vi "GPS_usb 파싱.vi"() -> ()   [LabVIEW 2020]
uses:
  <vilib>/Instr/_visa.llb/VISA Configure Serial Port (Instr).vi
panel:
  in  "탭 컨트롤":T1(tab)
  out "로그파일 데이터":cluster{"all rows":dbl[], "all rows":dbl[]}(graph)
  out "보간 데이터":cluster{"all rows":dbl[], "all rows":dbl[]}(graph)
  out "거리값 설정 데이터":cluster{"all rows":dbl[], "all rows":dbl[]}(graph)
  in  "로그 파일 경로":path
  in  "배수 설정":i32
  in  "거리 값":dbl=1.0 format="%#_13g"
  in  "로그 인덱스 선택(0)":i32
  in  "로그 인덱스 선택(1)":i32=1
  in  "보간 방법":i32(ring)=1 items=["최근접", "선형", "스플라인", "3차 에르미트", "라그랑지"]
  out "RMC":T2 {"Checksum" format="%x"}
  out "GGA":T3 {"Checksum" format="%x"}
  out "VTG":T4 {"Checksum" format="%x"}
  out "구좌표플롯":cluster{"배열":dbl[], "배열":dbl[]}(graph)
  out "평면좌표플롯":cluster{"배열":dbl[], "배열":dbl[]}(graph)
  out "버퍼 읽기":string
  out "도(Lat)":string
  out "도(Long)":string
  out "도분초(Long)":string
  out "도분초(Lat)":string
  out "Y(E)":dbl format="%#.6g"
  out "X(N)":dbl format="%#.6g"
  out "에러 출력":errorcluster
  in  "정지":bool
  in  "VISA name":refnum<visa-resource-name> caption="VISA 리소스 이름"
  in  "baud rate  2":u32=9600 caption="보 전송속도(9600)"
  in  "timeout":u32=10000 caption="타임아웃(10sec)"
  in  "에러 입력(에러 없음)":errorcluster
  out "결과 조향값":dbl format="%#_13g"
  in  "Ld":dbl
  in  "다음wp X값":dbl format="%#_13g"
  in  "GPS X값":dbl format="%#_13g"
  in  "다음wp Y값":dbl format="%#_13g"
  in  "GPS Y값":dbl format="%#_13g"
  in  "GPS 헤딩값":dbl format="%#_13g"
  in  "축거(m)":dbl=1.04 format="%#_13g"
  in  "시리얼 루프 정지":bool
  out "Receive Data":T5
  in  "E-Stop":enum8{"정상", "긴급정지"}(ring)
  in  "transmit Data":T6
  in  "시리얼 포트 설정":refnum<visa-resource-name> caption="VISA 리소스 이름"
  in  "baud rate":u32=9600 caption="보 전송속도(9600)"
  in  "timeout (100)":u32=10000 caption="타임아웃(10sec)"
  out "Lidar":cluster{"배열":dbl[], "배열":dbl[]}(graph)
  out "time stamp + factory":string
  in  "Lidar 정지":bool
  out "Mixed Signal Graph":cluster{dbl[], dbl[]}[](graph)
  out "Mixed Signal Graph 2":cluster{"array":dbl[], "array":dbl[]}[](graph)
  in  "점 개수":i32
  in  "사각형 크기 설정값":dbl
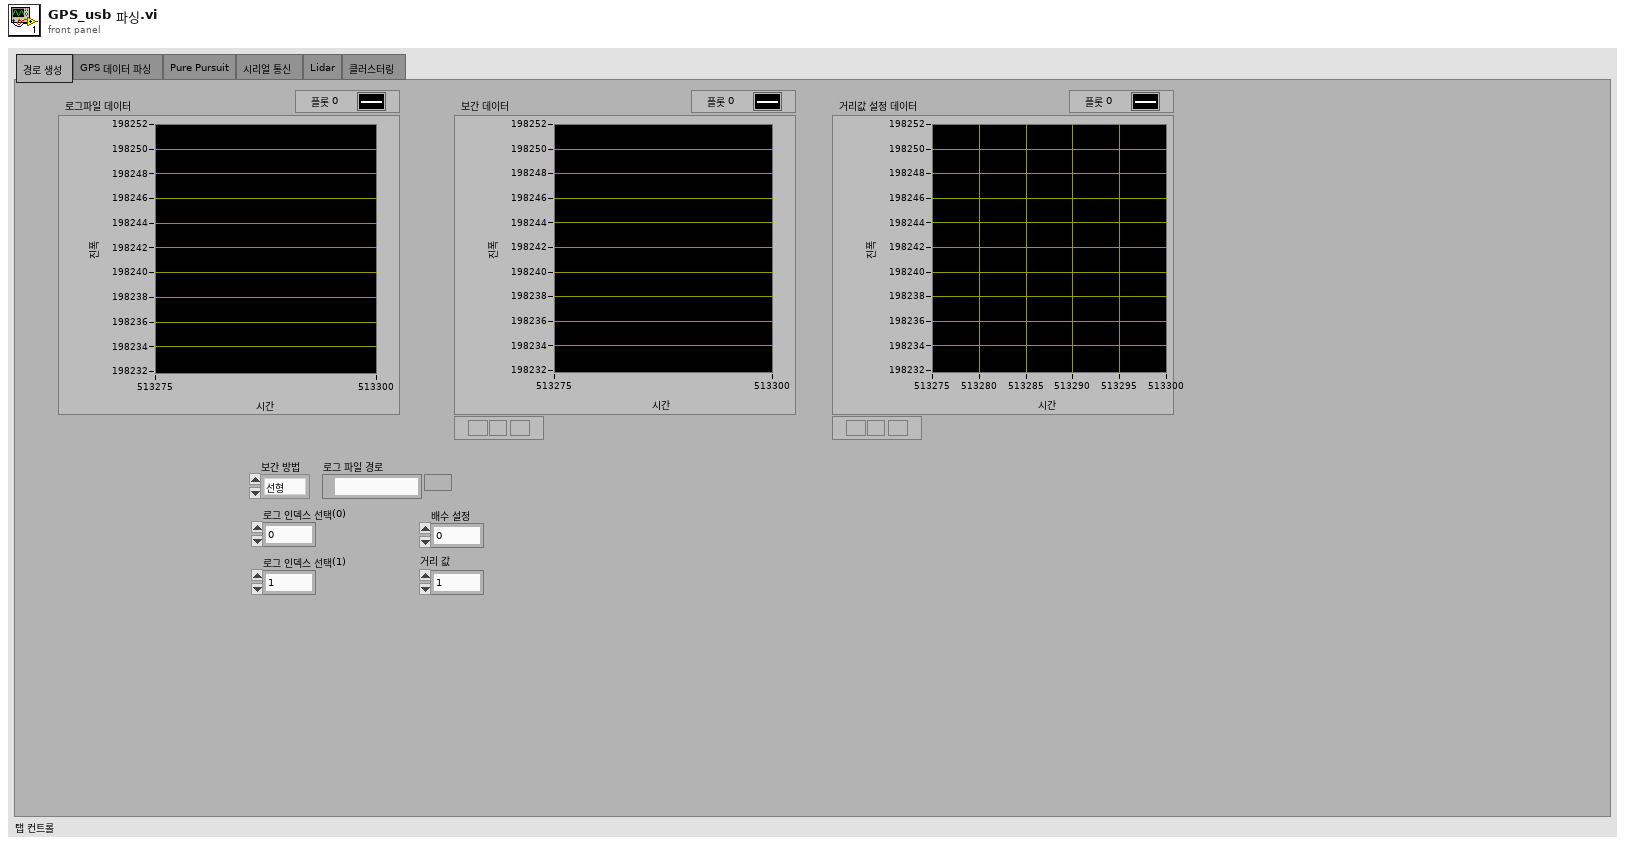
[diagram p1: front panel]
types:
  T1 = enum32{"경로 생성", "GPS 데이터 파싱", "Pure Pursuit", "시리얼 통신", "Lidar", "클러스터링"}
  T2 = cluster{"UTC time":dbl, "Status":string, "Latitude":dbl, "N/S Indicator":string, "Longitude":dbl, "E/W Indicator":string, "Speed":dbl, "Degrees":dbl, "UTC date":dbl, "Null":string, "Null 2":string, "Null 3":string, "Null 4":string, "Checksum":i32}
  T3 = cluster{"UTC time":dbl, "Latitude":dbl, "N/S Indicator":string, "Longitude":dbl, "E/W Indicator":string, "Position FIx":i32, "Satelites Used":i32, "HDOP":dbl, "Altitude":dbl, "Altitude Units":string, "empty":string, "empty":string, "empty":string, "Checksum":u8}
  T4 = cluster{"Course":dbl, "Reference":string, "Course in degrees":dbl, "Reference":string, "Speed":dbl, "Unit":string, "Speed":dbl, "K":string, "A":string, "Checksum":u8}
  T5 = cluster{"AorM":u8, "E-Stop":u8, "F_B":u8, "Speed":u16, "Steer":i16, "Brake":u8, "Encoder":u8, "Encoder2":u8, "Encoder3":u8, "Encoder4":u8, "ALIVE":u8, "ETX_0":u8, "ETX_1":u8}
  T6 = cluster{enum8{"Manual", "Auto"}, enum8{"전진", "중립", "후진"}, "Speed":u16, "Steer":i16, "Brake":u8}
  T7 = enum16{"open", "replace", "create", "open or create", "replace or create", "replace or create with confirmation"}
  T8 = cluster{"UTC time":dbl, "Status":string, "Latitude":dbl, "N/S Indicator":string, "Longitude":dbl, "E/W Indicator":string, "Speed":dbl, "Degrees":dbl, "UTC date":dbl, "Null":string, "Null 2":string, "Null 3":string, "Null 4":string, "Checksum":u8}
  T9 = cluster{"string array[0]":string, "string array[1]":string, "string array[2]":string, "string array[3]":string, "string array[4]":string, "string array[5]":string, "string array[6]":string, "string array[7]":string, "string array[8]":string, "string array[9]":string, "string array[10]":string, "string array[11]":string, "string array[12]":string}
  T10 = cluster{"string array[0]":string, "string array[1]":string, "string array[2]":string, "string array[3]":string, "string array[4]":string, "string array[5]":string, "string array[6]":string, "string array[7]":string, "string array[8]":string}
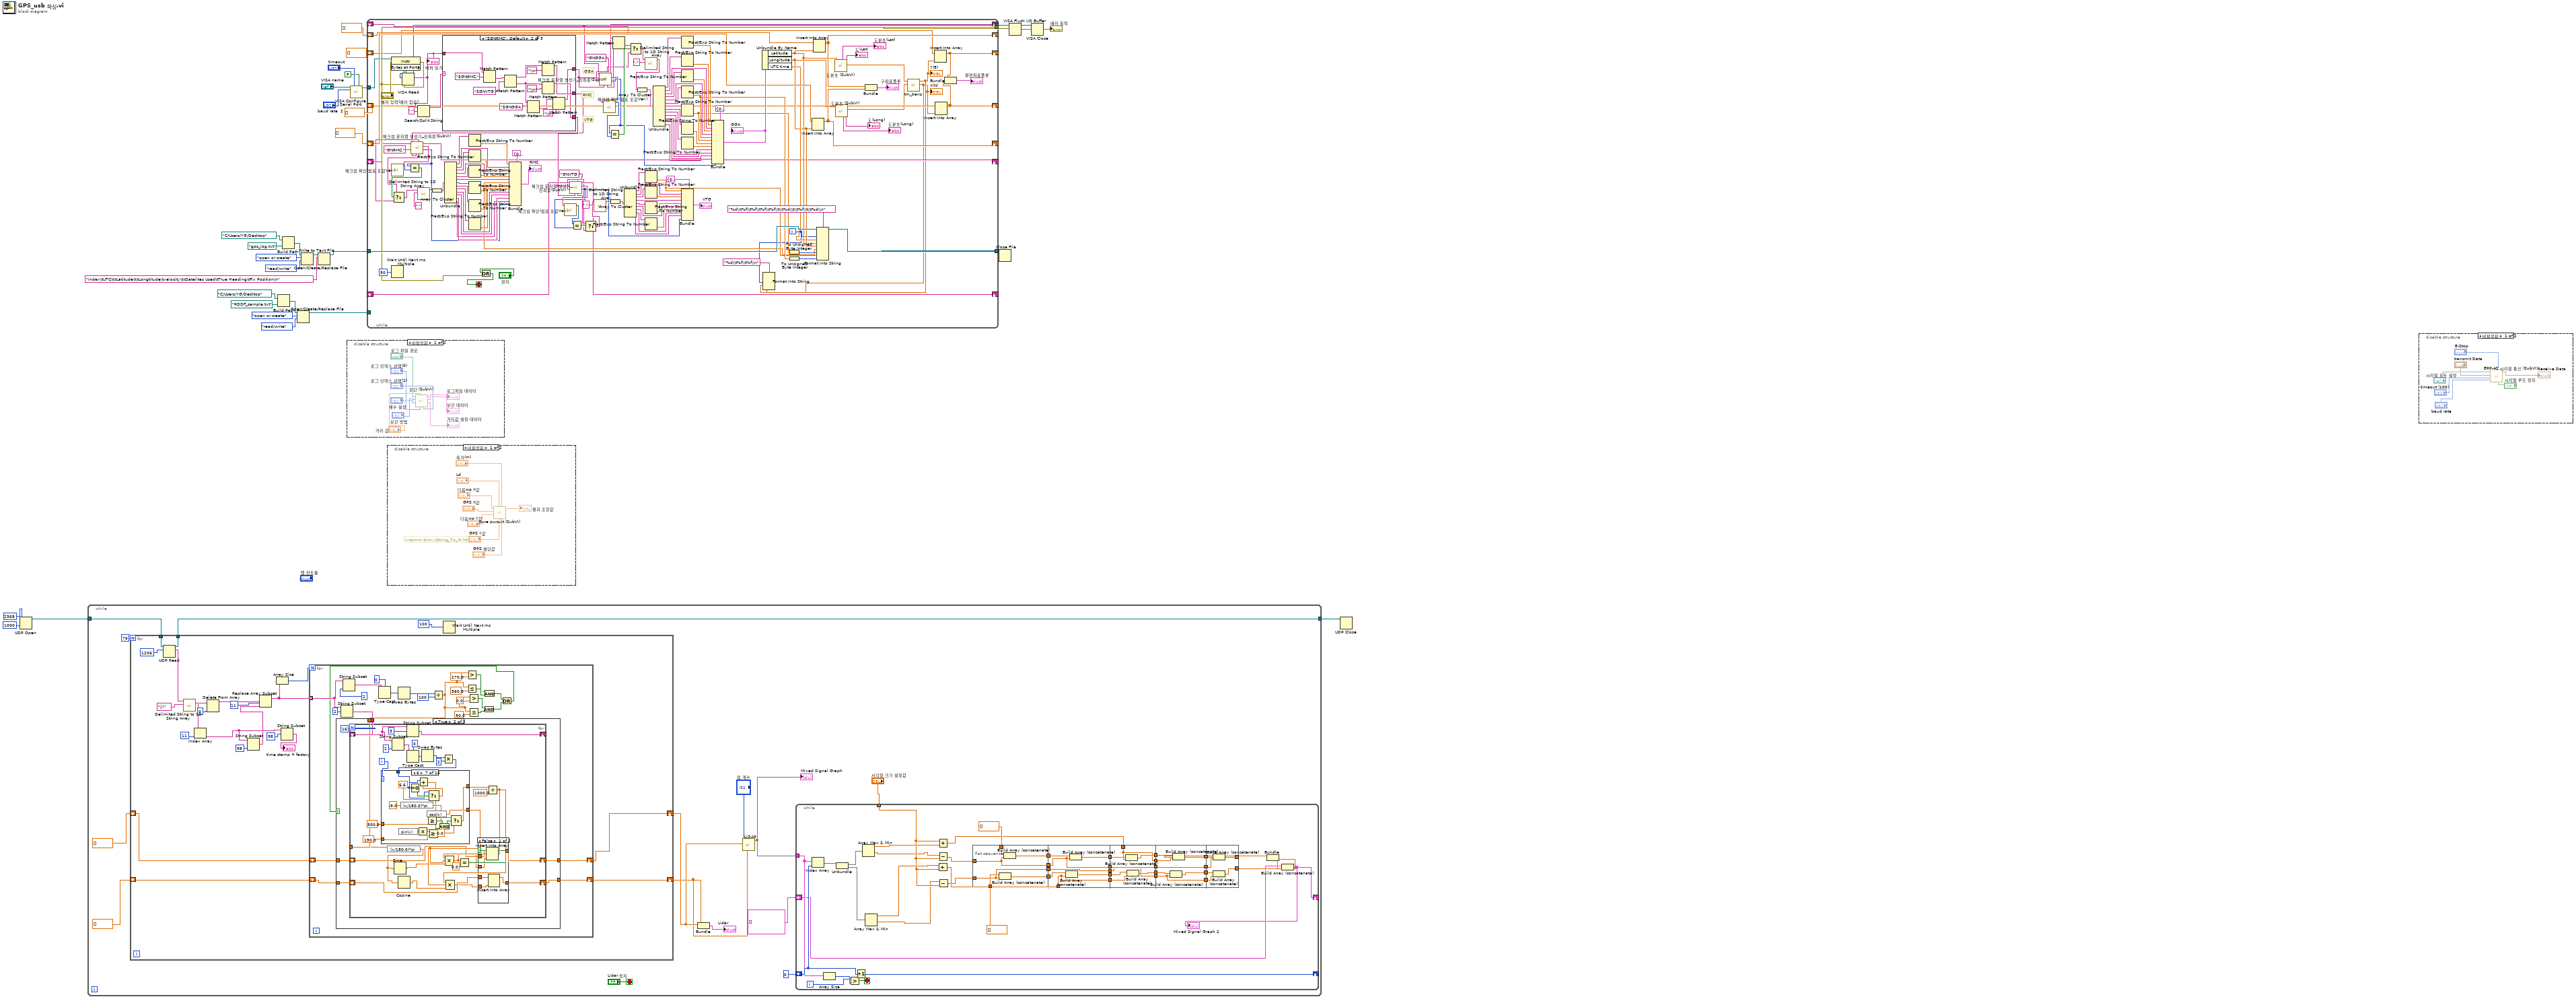
[diagram p0: block diagram]
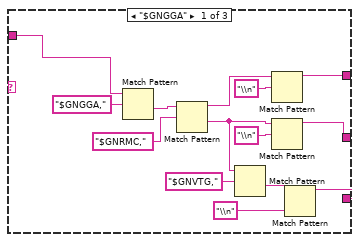
[diagram p2: hidden frame]
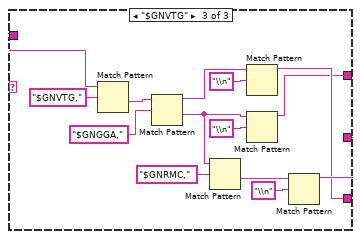
[diagram p3: hidden frame]
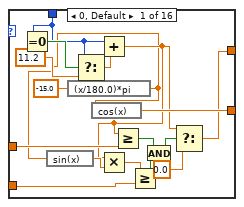
[diagram p6: hidden frame]
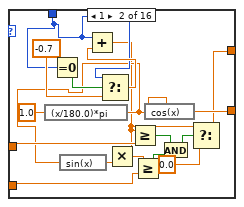
[diagram p7: hidden frame]
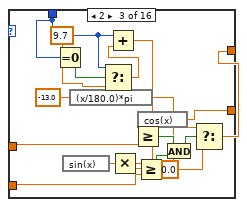
[diagram p8: hidden frame]
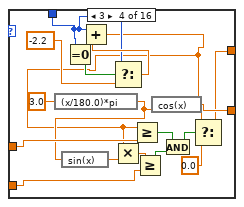
[diagram p9: hidden frame]
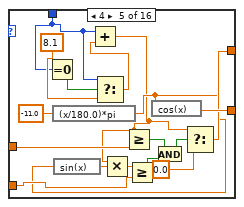
[diagram p10: hidden frame]
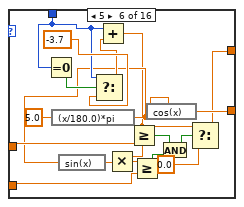
[diagram p11: hidden frame]
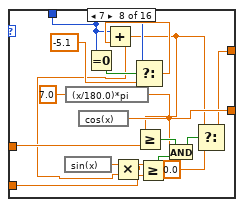
[diagram p12: hidden frame]
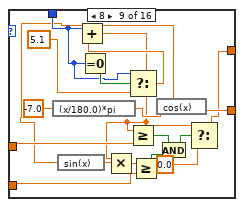
[diagram p13: hidden frame]
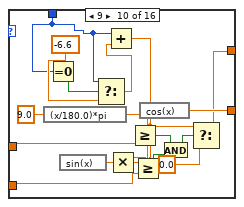
[diagram p14: hidden frame]
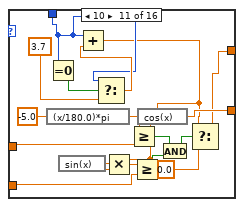
[diagram p15: hidden frame]
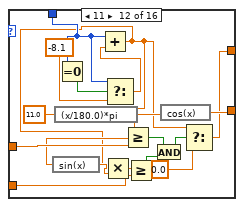
[diagram p16: hidden frame]
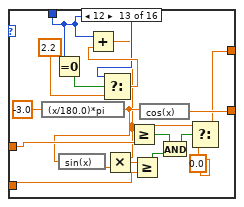
[diagram p17: hidden frame]
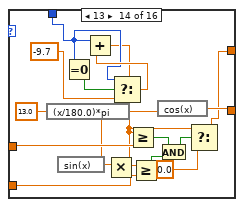
[diagram p18: hidden frame]
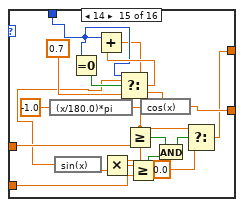
[diagram p19: hidden frame]
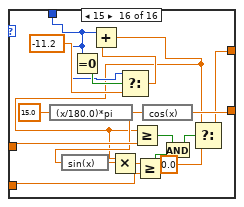
[diagram p20: hidden frame]
diagram:
  n1 = UDP Open(9:1000 ("타임아웃 ms (25000)"), 11:u16 2368 ("포트")) -> (port=w31:refnum<k16>)  [unwired: 3 in, 2 out]
  n2 = while {
    tunnel: w31 -> [w45]
    tunnel: [w44] -> w30
    stop <- "Lidar 정지" stop-if-true
    n3 = for {
      N: 76 -> [_]
      shift-right: [w127] -> w39
      shift-left: dbl[] [] -> [w132]
      shift-right: [w126] -> w38
      shift-left: dbl[] [] -> [w133]
      tunnel: w45 -> [w130]
      tunnel: [w128] -> w44
      n4 = UDP Read(connection ID=w130, max size (548)=1206 ("최대 크기(548)")) -> (data out=w129:string, 3:w128:refnum<k16>)  [unwired: 2 in, 3 out]
      n5 = call <vilib>:"Delimited String to 1D String Array.vi"("delimiter"="ÿî", "delimited string"=w129) -> ("string array"=w145:string[])  [unwired: 9 in]
      n6 = Delete From Array(array=w145, index=0 ("인덱스")) -> (array with subset deleted=w142:string[])  [unwired: 1 in, 1 out]
      n7 = Index Array(array=w142, index=11 ("인덱스")) -> (element=w138:string)
      n8 = String Subset(string=w138, length (rest)=98 ("길이(나머지)")) -> (substring=w137:string)  [unwired: 1 in]
      n9 = Replace Array Subset(array=w142, new element=w137, index=11 ("인덱스")) -> (w135:string[])
      n10 = Array Size(array=w135) -> (size(s)=w134:i32)
      n11 = String Subset(string=w138, offset (0)=98 ("오프셋(0)")) -> (substring=→"time stamp + factory":string)  [unwired: 1 in]
      n12 = for {
        N: w134 -> [_]
        tunnel: w135 -> [w164] mode=indexing
        shift-right: [w162] -> w126
        shift-left: w133 -> [w160]
        shift-right: [w161] -> w127
        shift-left: w132 -> [w159]
        n13 = String Subset(string=w164, offset (0)=2 ("오프셋(0)")) -> (substring=w163:string)  [unwired: 1 in]
        n14 = String Subset(string=w164, length (rest)=2 ("길이(나머지)")) -> (substring=w170:string)  [unwired: 1 in]
        n15 = Type Cast(type=u16 0, x=w170) -> (*(type *) &x=w168:u16)
        n16 = Swap Bytes(anything=w168) -> (byte swapped=w167:u16)
        n17 = Divide(x=w167, y=u16 100) -> (x/y=w152:dbl)
        n18 = Greater?(x=w152, y=270.0) -> (0:w155:bool)
        n19 = Less Or Equal?(x=w152, y=360.0) -> (x <= y?=w156:bool)
        n20 = Greater?(x=w152, y=0.0) -> (0:w151:bool)
        n21 = Less Or Equal?(x=w152, y=90.0) -> (x <= y?=w150:bool)
        n22 = And(x=w151, y=w150) -> (x .and. y?=w147:bool)
        n23 = And(x=w155, y=w156) -> (x .and. y?=w148:bool)
        n24 = Or(x=w148, y=w147) -> (x .or. y?=w149:bool)
        n25 = case shown="True" w149 {
          tunnel: w163 -> [_ w179]
          tunnel: w152 -> [_ w178]
          tunnel: [w172 w177] -> w162
          tunnel: [w173 w176] -> w161
          tunnel: w160 -> [w172 w175]
          tunnel: w159 -> [w173 w174]
          frame False {
          }
          frame True {
            n26 = for {
              N: 16 -> [_]
              shift-right: [w207] -> _
              shift-left: w179 -> [w206]
              tunnel: w178 -> [w199]
              shift-right: [w186] -> w176
              shift-left: w174 -> [w187]
              shift-right: [w183] -> w177
              shift-left: w175 -> [w184]
              i -> [w193]
              n27 = expression code="(x/180.0)*pi"(w199) -> (w195:dbl)
              n28 = String Subset(string=w206, length (rest)=u16 2 ("길이(나머지)")) -> (substring=w203:string)  [unwired: 1 in]
              n29 = Sine(x=w195) -> (sin(x)=w194:dbl)
              n30 = Cosine(x=w195) -> (cos(x)=w196:dbl)
              n31 = String Subset(string=w206, offset (0)=3 ("오프셋(0)")) -> (substring=w207:string)  [unwired: 1 in]
              n32 = Type Cast(type=u16 0, x=w203) -> (*(type *) &x=w204:u16)
              n33 = Swap Bytes(anything=w204) -> (byte swapped=w201:u16)
              n34 = Multiply(x=w201, y=u16 2 ("x")) -> (x*y=w200:u16)
              n35 = case shown="6" w193 {
                tunnel: w200 -> [w229 w246 w263 w280 w297 w314 w331 w348 w365 w382 w399 w416 w433 w450 w467 w484]
                tunnel: [w225 w239 w257 w274 w291 w308 w324 w341 w359 w376 w393 w409 w426 w444 w461 w478] -> w191
                tunnel: [w233 w250 w267 w284 w301 w318 w335 w352 w369 w386 w403 w420 w437 w454 w471 w488] -> w197
                tunnel: 500.0 ("거리 값(min)") -> [w224 w242 w259 w276 w293 w310 w327 w344 w361 w378 w395 w412 w428 w446 w463 w480]
                tunnel: 150.0 ("높이 값(min)") -> [w223 w241 w258 w275 w292 w309 w326 w343 w360 w377 w394 w411 w429 w445 w462 w479]
                frame 0, Default {
                  n36 = Equal To 0?(x=w229) -> (x = 0?=w231:bool)
                  n37 = expression code="(x/180.0)*pi"(-15.0) -> (w219:dbl)
                  n38 = expression code="sin(x)"(w219) -> (w221:dbl)
                  n39 = Select(t=w229, s=w231, f=11.2 ("y")) -> (s? t:f=w232:dbl)
                  n40 = expression code="cos(x)"(w219) -> (w233:dbl)
                  n41 = Add(x=w229, y=w232) -> (x+y=w220:dbl)
                  n42 = Multiply(x=w220, y=w221) -> (x*y=w222:dbl)
                  n43 = Greater Or Equal?(x=w220, y=w224) -> (x >= y?=w228:bool)
                  n44 = Greater Or Equal?(x=w222, y=w223) -> (x >= y?=w227:bool)
                  n45 = And(x=w228, y=w227) -> (x .and. y?=w226:bool)
                  n46 = Select(t=w220, s=w226, f=0.0) -> (s? t:f=w225:dbl)
                }
                frame 1 {
                  n47 = expression code="(x/180.0)*pi"(1.0) -> (w240:dbl)
                  n48 = Equal To 0?(x=w246) -> (x = 0?=w249:bool)
                  n49 = expression code="sin(x)"(w240) -> (w238:dbl)
                  n50 = Select(t=w246, s=w249, f=-0.7 ("y")) -> (s? t:f=w247:dbl)
                  n51 = Add(x=w246, y=w247) -> (x+y=w237:dbl)
                  n52 = Multiply(x=w237, y=w238) -> (x*y=w236:dbl)
                  n53 = Greater Or Equal?(x=w237, y=w242) -> (x >= y?=w245:bool)
                  n54 = Greater Or Equal?(x=w236, y=w241) -> (x >= y?=w244:bool)
                  n55 = expression code="cos(x)"(w240) -> (w250:dbl)
                  n56 = And(x=w245, y=w244) -> (x .and. y?=w243:bool)
                  n57 = Select(t=w237, s=w243, f=0.0) -> (s? t:f=w239:dbl)
                }
                frame 2 {
                  n58 = Equal To 0?(x=w263) -> (x = 0?=w266:bool)
                  n59 = expression code="(x/180.0)*pi"(-13.0) -> (w256:dbl)
                  n60 = expression code="sin(x)"(w256) -> (w255:dbl)
                  n61 = Select(t=w263, s=w266, f=9.7 ("y")) -> (s? t:f=w264:dbl)
                  n62 = Add(x=w263, y=w264) -> (x+y=w253:dbl)
                  n63 = Multiply(x=w255, y=w253) -> (x*y=w254:dbl)
                  n64 = Greater Or Equal?(x=w253, y=w259) -> (x >= y?=w262:bool)
                  n65 = Greater Or Equal?(x=w254, y=w258) -> (x >= y?=w261:bool)
                  n66 = expression code="cos(x)"(w256) -> (w267:dbl)
                  n67 = And(x=w262, y=w261) -> (x .and. y?=w260:bool)
                  n68 = Select(t=w253, s=w260, f=0.0) -> (s? t:f=w257:dbl)
                }
                frame 3 {
                  n69 = expression code="(x/180.0)*pi"(3.0) -> (w273:dbl)
                  n70 = expression code="sin(x)"(w273) -> (w272:dbl)
                  n71 = Equal To 0?(x=w280) -> (x = 0?=w283:bool)
                  n72 = Select(t=w280, s=w283, f=-2.2 ("y")) -> (s? t:f=w281:dbl)
                  n73 = Add(x=w280, y=w281) -> (x+y=w270:dbl)
                  n74 = Multiply(x=w270, y=w272) -> (x*y=w271:dbl)
                  n75 = Greater Or Equal?(x=w270, y=w276) -> (x >= y?=w279:bool)
                  n76 = Greater Or Equal?(x=w271, y=w275) -> (x >= y?=w278:bool)
                  n77 = expression code="cos(x)"(w273) -> (w284:dbl)
                  n78 = And(x=w279, y=w278) -> (x .and. y?=w277:bool)
                  n79 = Select(t=w270, s=w277, f=0.0) -> (s? t:f=w274:dbl)
                }
                frame 4 {
                  n80 = Equal To 0?(x=w297) -> (x = 0?=w300:bool)
                  n81 = expression code="(x/180.0)*pi"(-11.0) -> (w290:dbl)
                  n82 = expression code="sin(x)"(w290) -> (w289:dbl)
                  n83 = Select(t=w297, s=w300, f=8.1 ("y")) -> (s? t:f=w298:dbl)
                  n84 = Add(x=w297, y=w298) -> (x+y=w287:dbl)
                  n85 = Multiply(x=w287, y=w289) -> (x*y=w288:dbl)
                  n86 = Greater Or Equal?(x=w287, y=w293) -> (x >= y?=w296:bool)
                  n87 = Greater Or Equal?(x=w288, y=w292) -> (x >= y?=w295:bool)
                  n88 = expression code="cos(x)"(w290) -> (w301:dbl)
                  n89 = And(x=w296, y=w295) -> (x .and. y?=w294:bool)
                  n90 = Select(t=w287, s=w294, f=0.0) -> (s? t:f=w291:dbl)
                }
                frame 5 {
                  n91 = Equal To 0?(x=w314) -> (x = 0?=w317:bool)
                  n92 = expression code="(x/180.0)*pi"(5.0) -> (w307:dbl)
                  n93 = expression code="sin(x)"(w307) -> (w306:dbl)
                  n94 = Select(t=w314, s=w317, f=-3.7 ("y")) -> (s? t:f=w315:dbl)
                  n95 = Add(x=w314, y=w315) -> (x+y=w304:dbl)
                  n96 = Multiply(x=w304, y=w306) -> (x*y=w305:dbl)
                  n97 = Greater Or Equal?(x=w304, y=w310) -> (x >= y?=w313:bool)
                  n98 = Greater Or Equal?(x=w305, y=w309) -> (x >= y?=w312:bool)
                  n99 = expression code="cos(x)"(w307) -> (w318:dbl)
                  n100 = And(x=w313, y=w312) -> (x .and. y?=w311:bool)
                  n101 = Select(t=w304, s=w311, f=0.0) -> (s? t:f=w308:dbl)
                }
                frame 6 {
                  n102 = expression code="(x/180.0)*pi"(-9.0) -> (w325:dbl)
                  n103 = expression code="sin(x)"(w325) -> (w322:dbl)
                  n104 = Equal To 0?(x=w331) -> (x = 0?=w334:bool)
                  n105 = expression code="cos(x)"(w325) -> (w335:dbl)
                  n106 = Select(t=w331, s=w334, f=6.6 ("y")) -> (s? t:f=w332:dbl)
                  n107 = Add(x=w331, y=w332) -> (x+y=w321:dbl)
                  n108 = Multiply(x=w321, y=w322) -> (x*y=w323:dbl)
                  n109 = Greater Or Equal?(x=w321, y=w327) -> (x >= y?=w330:bool)
                  n110 = Greater Or Equal?(x=w323, y=w326) -> (x >= y?=w329:bool)
                  n111 = And(x=w330, y=w329) -> (x .and. y?=w328:bool)
                  n112 = Select(t=w321, s=w328, f=0.0) -> (s? t:f=w324:dbl)
                }
                frame 7 {
                  n113 = expression code="(x/180.0)*pi"(7.0) -> (w342:dbl)
                  n114 = expression code="sin(x)"(w342) -> (w340:dbl)
                  n115 = expression code="cos(x)"(w342) -> (w352:dbl)
                  n116 = Equal To 0?(x=w348) -> (x = 0?=w351:bool)
                  n117 = Select(t=w348, s=w351, f=-5.1 ("y")) -> (s? t:f=w349:dbl)
                  n118 = Add(x=w348, y=w349) -> (x+y=w339:dbl)
                  n119 = Multiply(x=w340, y=w339) -> (x*y=w338:dbl)
                  n120 = Greater Or Equal?(x=w339, y=w344) -> (x >= y?=w347:bool)
                  n121 = Greater Or Equal?(x=w338, y=w343) -> (x >= y?=w346:bool)
                  n122 = And(x=w347, y=w346) -> (x .and. y?=w345:bool)
                  n123 = Select(t=w339, s=w345, f=0.0) -> (s? t:f=w341:dbl)
                }
                frame 8 {
                  n124 = expression code="(x/180.0)*pi"(-7.0) -> (w358:dbl)
                  n125 = expression code="sin(x)"(w358) -> (w357:dbl)
                  n126 = Equal To 0?(x=w365) -> (x = 0?=w368:bool)
                  n127 = Select(t=w365, s=w368, f=5.1 ("y")) -> (s? t:f=w366:dbl)
                  n128 = Add(x=w365, y=w366) -> (x+y=w355:dbl)
                  n129 = Multiply(x=w355, y=w357) -> (x*y=w356:dbl)
                  n130 = Greater Or Equal?(x=w355, y=w361) -> (x >= y?=w364:bool)
                  n131 = Greater Or Equal?(x=w356, y=w360) -> (x >= y?=w363:bool)
                  n132 = expression code="cos(x)"(w358) -> (w369:dbl)
                  n133 = And(x=w364, y=w363) -> (x .and. y?=w362:bool)
                  n134 = Select(t=w355, s=w362, f=0.0) -> (s? t:f=w359:dbl)
                }
                frame 9 {
                  n135 = expression code="(x/180.0)*pi"(9.0) -> (w375:dbl)
                  n136 = Equal To 0?(x=w382) -> (x = 0?=w385:bool)
                  n137 = expression code="sin(x)"(w375) -> (w374:dbl)
                  n138 = Select(t=w382, s=w385, f=-6.6 ("y")) -> (s? t:f=w383:dbl)
                  n139 = Add(x=w382, y=w383) -> (x+y=w372:dbl)
                  n140 = Multiply(x=w372, y=w374) -> (x*y=w373:dbl)
                  n141 = Greater Or Equal?(x=w372, y=w378) -> (x >= y?=w381:bool)
                  n142 = Greater Or Equal?(x=w373, y=w377) -> (x >= y?=w380:bool)
                  n143 = expression code="cos(x)"(w375) -> (w386:dbl)
                  n144 = And(x=w381, y=w380) -> (x .and. y?=w379:bool)
                  n145 = Select(t=w372, s=w379, f=0.0) -> (s? t:f=w376:dbl)
                }
                frame 10 {
                  n146 = expression code="(x/180.0)*pi"(-5.0) -> (w389:dbl)
                  n147 = Equal To 0?(x=w399) -> (x = 0?=w402:bool)
                  n148 = expression code="sin(x)"(w389) -> (w390:dbl)
                  n149 = Select(t=w399, s=w402, f=3.7 ("y")) -> (s? t:f=w400:dbl)
                  n150 = Add(x=w399, y=w400) -> (x+y=w392:dbl)
                  n151 = Multiply(x=w389, y=w390) -> (x*y=w391:dbl)
                  n152 = Greater Or Equal?(x=w392, y=w395) -> (x >= y?=w398:bool)
                  n153 = Greater Or Equal?(x=w391, y=w394) -> (x >= y?=w397:bool)
                  n154 = expression code="cos(x)"(w389) -> (w403:dbl)
                  n155 = And(x=w398, y=w397) -> (x .and. y?=w396:bool)
                  n156 = Select(t=w392, s=w396, f=0.0) -> (s? t:f=w393:dbl)
                }
                frame 11 {
                  n157 = expression code="(x/180.0)*pi"(11.0) -> (w410:dbl)
                  n158 = expression code="sin(x)"(w410) -> (w408:dbl)
                  n159 = Equal To 0?(x=w416) -> (x = 0?=w419:bool)
                  n160 = Select(t=w416, s=w419, f=-8.1 ("y")) -> (s? t:f=w417:dbl)
                  n161 = Add(x=w416, y=w417) -> (x+y=w406:dbl)
                  n162 = Multiply(x=w406, y=w408) -> (x*y=w407:dbl)
                  n163 = Greater Or Equal?(x=w406, y=w412) -> (x >= y?=w415:bool)
                  n164 = Greater Or Equal?(x=w407, y=w411) -> (x >= y?=w414:bool)
                  n165 = And(x=w415, y=w414) -> (x .and. y?=w413:bool)
                  n166 = expression code="cos(x)"(w410) -> (w420:dbl)
                  n167 = Select(t=w406, s=w413, f=0.0) -> (s? t:f=w409:dbl)
                }
                frame 12 {
                  n168 = expression code="(x/180.0)*pi"(-3.0) -> (w427:dbl)
                  n169 = Equal To 0?(x=w433) -> (x = 0?=w436:bool)
                  n170 = expression code="sin(x)"(w427) -> (w424:dbl)
                  n171 = Select(t=w433, s=w436, f=2.2 ("y")) -> (s? t:f=w434:dbl)
                  n172 = Add(x=w433, y=w434) -> (x+y=w423:dbl)
                  n173 = Multiply(x=w423, y=w424) -> (x*y=w425:dbl)
                  n174 = Greater Or Equal?(x=w423, y=w428) -> (x >= y?=w432:bool)
                  n175 = Greater Or Equal?(x=w425, y=w429) -> (x >= y?=w431:bool)
                  n176 = expression code="cos(x)"(w427) -> (w437:dbl)
                  n177 = And(x=w432, y=w431) -> (x .and. y?=w430:bool)
                  n178 = Select(t=w423, s=w430, f=0.0) -> (s? t:f=w426:dbl)
                }
                frame 13 {
                  n179 = expression code="(x/180.0)*pi"(13.0) -> (w443:dbl)
                  n180 = expression code="sin(x)"(w443) -> (w441:dbl)
                  n181 = Equal To 0?(x=w450) -> (x = 0?=w453:bool)
                  n182 = Select(t=w450, s=w453, f=-9.7 ("y")) -> (s? t:f=w451:dbl)
                  n183 = Add(x=w450, y=w451) -> (x+y=w440:dbl)
                  n184 = Multiply(x=w440, y=w441) -> (x*y=w442:dbl)
                  n185 = Greater Or Equal?(x=w440, y=w446) -> (x >= y?=w449:bool)
                  n186 = Greater Or Equal?(x=w442, y=w445) -> (x >= y?=w448:bool)
                  n187 = expression code="cos(x)"(w443) -> (w454:dbl)
                  n188 = And(x=w449, y=w448) -> (x .and. y?=w447:bool)
                  n189 = Select(t=w440, s=w447, f=0.0) -> (s? t:f=w444:dbl)
                }
                frame 14 {
                  n190 = expression code="(x/180.0)*pi"(-1.0) -> (w460:dbl)
                  n191 = expression code="sin(x)"(w460) -> (w459:dbl)
                  n192 = Equal To 0?(x=w467) -> (x = 0?=w470:bool)
                  n193 = Select(t=w467, s=w470, f=0.7 ("y")) -> (s? t:f=w468:dbl)
                  n194 = Add(x=w467, y=w468) -> (x+y=w457:dbl)
                  n195 = Multiply(x=w457, y=w459) -> (x*y=w458:dbl)
                  n196 = Greater Or Equal?(x=w457, y=w463) -> (x >= y?=w466:bool)
                  n197 = Greater Or Equal?(x=w458, y=w462) -> (x >= y?=w465:bool)
                  n198 = expression code="cos(x)"(w460) -> (w471:dbl)
                  n199 = And(x=w466, y=w465) -> (x .and. y?=w464:bool)
                  n200 = Select(t=w457, s=w464, f=0.0) -> (s? t:f=w461:dbl)
                }
                frame 15 {
                  n201 = expression code="(x/180.0)*pi"(15.0) -> (w477:dbl)
                  n202 = expression code="sin(x)"(w477) -> (w476:dbl)
                  n203 = Equal To 0?(x=w484) -> (x = 0?=w487:bool)
                  n204 = Select(t=w484, s=w487, f=-11.2 ("y")) -> (s? t:f=w485:dbl)
                  n205 = Add(x=w484, y=w485) -> (x+y=w474:dbl)
                  n206 = Multiply(x=w474, y=w476) -> (x*y=w475:dbl)
                  n207 = Greater Or Equal?(x=w474, y=w480) -> (x >= y?=w483:bool)
                  n208 = Greater Or Equal?(x=w475, y=w479) -> (x >= y?=w482:bool)
                  n209 = expression code="cos(x)"(w477) -> (w488:dbl)
                  n210 = And(x=w483, y=w482) -> (x .and. y?=w481:bool)
                  n211 = Select(t=w474, s=w481, f=0.0) -> (s? t:f=w478:dbl)
                }
              }
              n212 = Divide(x=w191, y=1000.0) -> (x/y=w192:dbl)
              n213 = Compound Arithmetic op=MULTIPLY(w192, w197, w194) -> (w181:dbl)
              n214 = Compound Arithmetic op=MULTIPLY(w192, w197, w196) -> (w182:dbl)
              n215 = Equal?(x=w181, y=0.0) -> (x = y?=w188:bool)
              n216 = case shown="False" w188 {
                tunnel: w187 -> [w215 w217]
                tunnel: [w210 w217] -> w186
                tunnel: w181 -> [w214 _]
                tunnel: w184 -> [w213 w216]
                tunnel: [w212 w216] -> w183
                tunnel: w182 -> [w211 _]
                frame False {
                  n217 = Insert Into Array(array=w215, new element=w214) -> (w210:dbl[])  [unwired: 1 in]
                  n218 = Insert Into Array(array=w213, new element=w211) -> (w212:dbl[])  [unwired: 1 in]
                }
                frame True {
                }
              }
            }
          }
        }
      }
    }
    n219 = Wait Until Next ms Multiple(millisecond multiple=u32 100 ("ms 배수")) -> ()  [unwired: 1 out]
    n220 = Bundle(w39, w38) -> (→"Lidar":cluster{dbl[], dbl[]})  [unwired: 1 in]
    n221 = call "LiDAR.vi"(6:w38, 10:w39, 11:"점 개수") -> (3:w34)  [unwired: 8 in]
    "Mixed Signal Graph" <- w34
    n222 = while {
      shift-right: [w91] -> _
      shift-left: 0 ("인덱스") -> [w90]
      tunnel: w34 -> [w89]
      tunnel: "사각형 크기 설정값" -> [w84]
      shift-right: [w55] -> _
      shift-left: cluster{dbl[], dbl[]}[] [] ("배열") -> [w56]
      i -> [w88]
      stop <- w86 stop-if-true
      n223 = Index Array(array=w89, index=w90) -> (element=w85)
      n224 = Array Size(array=w89) -> (size(s)=w87:i32)
      n225 = Unbundle(w85) -> (w51, w54)
      n226 = Greater?(x=w88, y=w87) -> (0:w86:bool)
      n227 = Increment(x=w90) -> (x+1=w91:i32)
      n228 = Array Max & Min(array=w51) -> (max value=w50:dbl, min value=w49:dbl)  [unwired: 2 out]
      n229 = Array Max & Min(array=w54) -> (max value=w53:dbl, min value=w52:dbl)  [unwired: 2 out]
      n230 = Add(x=w53, y=w84) -> (x+y=w70:dbl)
      n231 = Add(x=w84, y=w50) -> (x+y=w77:dbl)
      n232 = Subtract(x=w49, y=w84) -> (x-y=w82:dbl)
      n233 = Subtract(x=w52, y=w84) -> (x-y=w71:dbl)
      n234 = flat-sequence {
        tunnel: w82 -> [w96]
        tunnel: [w97] -> w83
        tunnel: [w96] -> w81
        tunnel: dbl[] [] ("배열") -> [w95]
        tunnel: w71 -> [w94]
        tunnel: [w94] -> w66
        tunnel: [w93] -> w64
        tunnel: dbl[] [] ("배열") -> [w92]
        tunnel: w83 -> [w104]
        tunnel: w81 -> [w102]
        tunnel: [w103] -> w80
        tunnel: [w102] -> w72
        tunnel: w70 -> [w101]
        tunnel: [w101] -> w69
        tunnel: [w100] -> w67
        tunnel: w66 -> [w100]
        tunnel: w64 -> [w99]
        tunnel: [w98] -> w63
        tunnel: w80 -> [w112]
        tunnel: [w111] -> w79
        tunnel: w77 -> [w110]
        tunnel: [w110] -> w76
        tunnel: [w109] -> w73
        tunnel: w72 -> [w109]
        tunnel: w69 -> [w108]
        tunnel: [w107] -> w68
        tunnel: w67 -> [w107]
        tunnel: w63 -> [w106]
        tunnel: [w105] -> w62
        tunnel: w79 -> [w119]
        tunnel: w76 -> [w118]
        tunnel: [w117] -> w75
        tunnel: [w116] -> w74
        tunnel: w73 -> [w116]
        tunnel: w68 -> [w115]
        tunnel: [w115] -> w65
        tunnel: w62 -> [w114]
        tunnel: [w113] -> w61
        tunnel: w75 -> [w125]
        tunnel: w74 -> [w124]
        tunnel: w65 -> [w123]
        tunnel: w61 -> [w122]
        tunnel: [w121] -> w59
        tunnel: [w120] -> w58
        frame #0 {
          n235 = Build Array (concatenate)(w92, w94) -> (w93:dbl[])
          n236 = Build Array (concatenate)(w95, w96) -> (w97:dbl[])
        }
        frame #1 {
          n237 = Build Array (concatenate)(w99, w101) -> (w98:dbl[])
          n238 = Build Array (concatenate)(w104, w102) -> (w103:dbl[])
        }
        frame #2 {
          n239 = Build Array (concatenate)(w112, w110) -> (w111:dbl[])
          n240 = Build Array (concatenate)(w106, w108) -> (w105:dbl[])
        }
        frame #3 {
          n241 = Build Array (concatenate)(w114, w115) -> (w113:dbl[])
          n242 = Build Array (concatenate)(w119, w118) -> (w117:dbl[])
        }
        frame #4 {
          n243 = Build Array (concatenate)(w125, w124) -> (w121:dbl[])
          n244 = Build Array (concatenate)(w122, w123) -> (w120:dbl[])
        }
      }
      n245 = Bundle(w59, w58) -> (w57:cluster{dbl[], dbl[]})  [unwired: 1 in]
      n246 = Build Array (concatenate)(w56, w57) -> (w55:cluster{dbl[], dbl[]}[])
      "Mixed Signal Graph 2" <- w55
    }
  }
  n247 = Build Path(base path=path "C:/Users/YG/Desktop" ("베이스 경로"), name or relative path=path "RDDF_sample.txt" ("이름 또는 상대 경로")) -> (appended path=w6:path)
  n248 = Build Path(base path=path "C:/Users/YG/Desktop" ("베이스 경로"), name or relative path=path "gps_log.txt" ("이름 또는 상대 경로")) -> (appended path=w26:path)
  n249 = Open/Create/Replace File(file path (use dialog)=w6, operation (0:open)=T7."open or create" ("동작(0:open)"), access (0:read/write)=enum16{"read/write", "read-only", "write-only"}."read/write" ("접근(0:읽기/쓰기)")) -> (refnum out=w1:refnum<file>)  [unwired: 3 in, 2 out]
  n250 = Open/Create/Replace File(file path (use dialog)=w26, operation (0:open)=T7."open or create" ("동작(0:open)"), access (0:read/write)=enum16{"read/write", "read-only", "write-only"}."read/write" ("접근(0:읽기/쓰기)")) -> (refnum out=w27:refnum<file>)  [unwired: 3 in, 2 out]
  n251 = Write to Text File(file (use dialog)=w27, text="Index\tUTC\t\tLatitude\t\tLongtitude\tvelocity\t\tSatelites Used\tTrue Heading\tFix Position\n" ("텍스트")) -> (refnum out=w9:refnum<file>)  [unwired: 2 in, 2 out]
  n252 = disable-structure shown="비활성화" {
    frame Disabled {
      n253 = call "보간 (SubVI).vi"("로그 인덱스 선택(1)"="로그 인덱스 선택(1)", "로그 인덱스 선택(0)"="로그 인덱스 선택(0)", "거리 상한 값"="거리 값", "배수 설정"="배수 설정", "보간 방법"="보간 방법", "로그 파일 경로"="로그 파일 경로") -> ("거리값 설정 데이터"=→"거리값 설정 데이터":cluster{"all rows":dbl[], "all rows":dbl[]}, "로그파일 데이터"=→"로그파일 데이터":cluster{"all rows":dbl[], "all rows":dbl[]}, "보간 데이터"=→"보간 데이터":cluster{"all rows":dbl[], "all rows":dbl[]})  [unwired: 3 in]
    }
    frame Enabled {
    }
  }
  n254 = call-poly "VISA Configure Serial Port"("VISA resource name"="VISA name", "timeout (10sec)"="timeout", "Enable Termination\nChar (T)"=FALSE ("Enable Termination\nChar (T)"), "baud rate (9600)"="baud rate  2") -> ("VISA resource name out"=w17:refnum<visa-resource-name>)  [unwired: 10 in, 1 out]
  n255 = while {
    shift-right: [w586] -> _
    shift-left: dbl[] [] ("배열") -> [w585]
    shift-right: [w587] -> _
    shift-left: dbl[] [] ("배열") -> [w584]
    tunnel: w17 -> [w567]
    tunnel: [w564] -> w14
    tunnel: [w560] -> w13
    tunnel: w9 -> [w580]
    tunnel: [w572] -> w21
    shift-right: [w508] -> _
    shift-left: _ -> [w509]
    shift-right: [w513] -> _
    shift-left: _ -> [w511]
    shift-right: [w514] -> _
    shift-left: _ -> [w510]
    shift-right: [w527] -> _
    shift-left: dbl[] [] -> [w529]
    shift-right: [w528] -> _
    shift-left: dbl[] [] -> [w530]
    tunnel: w1 -> [_]
    i -> [w502]
    stop <- w582 stop-if-true
    # "VTG"
    # "RMC"
    # "GGA"
    n256 = property class="Instr"(reference=w567, error in="에러 입력(에러 없음)") -> (reference out=w566:refnum<visa-resource-name>, error out=w561:errorcluster, "Bytes at Port"=w563:u32)
    n257 = Wait Until Next ms Multiple(millisecond multiple=u32 50 ("ms 배수")) -> ()  [unwired: 1 out]
    n258 = VISA Read(VISA resource name=w566, byte count=w563, error in (no error)=w561) -> (VISA resource name out=w564:refnum<visa-resource-name>, read buffer=w552:string, error out=w560:errorcluster)  [unwired: 1 out]
    "버퍼 읽기" <- w552
    n259 = Search/Split String(string=w552, search string/char (-)="," ("검색 문자열/문자 (-)")) -> (substring before match=w554:string)  [unwired: 1 in, 2 out]
    n260 = case shown="\"$GNRMC\", Default" w554 {
      tunnel: w552 -> [w643 w657 w671]
      tunnel: [w642 w654 w668] -> w543
      tunnel: [w641 w655 w669] -> w534
      tunnel: [w640 w656 w670] -> w521
      frame "$GNGGA" {
        n261 = Match Pattern(string=w643, regular expression="$GNGGA," ("정규식")) -> (after substring=w651:string)  [unwired: 1 in, 3 out]
        n262 = Match Pattern(string=w651, regular expression="$GNRMC," ("정규식")) -> (before substring=w645:string, after substring=w649:string)  [unwired: 1 in, 2 out]
        n263 = Match Pattern(string=w649, regular expression="$GNVTG," ("정규식")) -> (after substring=w647:string)  [unwired: 1 in, 3 out]
        n264 = Match Pattern(string=w645, regular expression="\\n" ("정규식")) -> (before substring=w642:string)  [unwired: 1 in, 3 out]
        n265 = Match Pattern(string=w649, regular expression="\\n" ("정규식")) -> (before substring=w640:string)  [unwired: 1 in, 3 out]
        n266 = Match Pattern(string=w647, regular expression="\\n" ("정규식")) -> (before substring=w641:string)  [unwired: 1 in, 3 out]
      }
      frame "$GNRMC", Default {
        n267 = Match Pattern(string=w657, regular expression="$GNRMC," ("정규식")) -> (after substring=w665:string)  [unwired: 1 in, 3 out]
        n268 = Match Pattern(string=w665, regular expression="$GNVTG," ("정규식")) -> (before substring=w659:string, after substring=w663:string)  [unwired: 1 in, 2 out]
        n269 = Match Pattern(string=w663, regular expression="$GNGGA," ("정규식")) -> (after substring=w661:string)  [unwired: 1 in, 3 out]
        n270 = Match Pattern(string=w659, regular expression="\\n" ("정규식")) -> (before substring=w656:string)  [unwired: 1 in, 3 out]
        n271 = Match Pattern(string=w663, regular expression="\\n" ("정규식")) -> (before substring=w655:string)  [unwired: 1 in, 3 out]
        n272 = Match Pattern(string=w661, regular expression="\\n" ("정규식")) -> (before substring=w654:string)  [unwired: 1 in, 3 out]
      }
      frame "$GNVTG" {
        n273 = Match Pattern(string=w671, regular expression="$GNVTG," ("정규식")) -> (after substring=w679:string)  [unwired: 1 in, 3 out]
        n274 = Match Pattern(string=w679, regular expression="$GNGGA," ("정규식")) -> (before substring=w673:string, after substring=w677:string)  [unwired: 1 in, 2 out]
        n275 = Match Pattern(string=w677, regular expression="$GNRMC," ("정규식")) -> (after substring=w675:string)  [unwired: 1 in, 3 out]
        n276 = Match Pattern(string=w673, regular expression="\\n" ("정규식")) -> (before substring=w669:string)  [unwired: 1 in, 3 out]
        n277 = Match Pattern(string=w677, regular expression="\\n" ("정규식")) -> (before substring=w668:string)  [unwired: 1 in, 3 out]
        n278 = Match Pattern(string=w675, regular expression="\\n" ("정규식")) -> (before substring=w670:string)  [unwired: 1 in, 3 out]
      }
    }
    n279 = call "체크섬 문자열 생성기_진최종(SubVI).vi"("raw data 입력"=w521, "GPS ID 입력"="GNRMC," ("GPS ID"), "입력 문자열 입력"=w521, "시프트레지스터(이전값) 입력 입력"=w511) -> ("숫자"=w520:u8, "checksum 확인용 문자열 2"=w523:string, "시프트레지스터용 출력 문자열"=w513:string, "클러스터 분배용 문자열 2"=w512:string, "클러스터 분배용 시프트레지스터"=w504:string)  [unwired: 3 in]
    n280 = call "체크섬 확인(쉼표 포함Ver.).vi"("입력 문자열"=w523) -> ("Checksum 비교값"=w539:u8)  [unwired: 10 in]
    n281 = Equal?(x=w520, y=w539) -> (x = y?=w538:bool)
    n282 = Select(t=w512, s=w538, f=w504) -> (s? t:f=w522:string)
    n283 = call <vilib>:"Delimited String to 1D String Array.vi"("delimiter"=",", "delimited string"=w522) -> ("string array"=w607:string[])  [unwired: 9 in]
    n284 = Array To Cluster(array=w607) -> (cluster=w605:T9)
    n285 = Unbundle(w605) -> ("string array[0]"=w609:string, "string array[1]"=w610:string, "string array[2]"=w611:string, "string array[3]"=w612:string, "string array[4]"=w613:string, "string array[5]"=w614:string, "string array[6]"=w615:string, "string array[7]"=w616:string, "string array[8]"=w617:string, "string array[9]"=w619:string, "string array[10]"=w604:string, "string array[11]"=w551:string, "string array[12]"=w525:string)
    n286 = Fract/Exp String To Number(string=w609) -> (number=w570:dbl)  [unwired: 3 in, 1 out]
    n287 = Fract/Exp String To Number(string=w611) -> (number=w569:dbl)  [unwired: 3 in, 1 out]
    n288 = Fract/Exp String To Number(string=w613) -> (number=w568:dbl)  [unwired: 3 in, 1 out]
    n289 = Fract/Exp String To Number(string=w615) -> (number=w555:dbl)  [unwired: 3 in, 1 out]
    n290 = Fract/Exp String To Number(string=w616) -> (number=w574:dbl)  [unwired: 3 in, 1 out]
    n291 = Fract/Exp String To Number(string=w617) -> (number=w618:dbl)  [unwired: 3 in, 1 out]
    n292 = Or(x="정지", y=w560) -> (x .or. y?=w582:bool)
    n293 = Bundle(cluster=T8 {"UTC time"=0.0, "Status"="", "Latitude"=0.0, "N/S Indicator"="", "Longitude"=0.0, "E/W Indicator"="", "Speed"=0.0, "Degrees"=0.0, "UTC date"=0.0, "Null"="", "Null 2"="", "Null 3"="", "Null 4"="", "Checksum"=0}, "UTC time"=w570, "Status"=w610, "Latitude"=w569, "N/S Indicator"=w612, "Longitude"=w568, "E/W Indicator"=w614, "Speed"=w555, "Degrees"=w574, "UTC date"=w618, "Null"=w619, "Null 2"=w604, "Null 3"=w551, "Null 4"=w525, "Checksum"=w520) -> (→"RMC":T8)
    n294 = call "체크섬 문자열 생성기_진최종(SubVI).vi"("raw data 입력"=w534, "GPS ID 입력"="GNVTG," ("GPS ID"), "입력 문자열 입력"=w534, "시프트레지스터(이전값) 입력 입력"=w510) -> ("숫자"=w516:u8, "checksum 확인용 문자열 2"=w535:string, "시프트레지스터용 출력 문자열"=w514:string, "클러스터 분배용 문자열 2"=w531:string, "클러스터 분배용 시프트레지스터"=w503:string)  [unwired: 3 in]
    n295 = call "체크섬 확인(쉼표 포함Ver.).vi"("입력 문자열"=w535) -> ("Checksum 비교값"=w537:u8)  [unwired: 10 in]
    n296 = Equal?(x=w537, y=w516) -> (x = y?=w536:bool)
    n297 = Select(t=w531, s=w536, f=w503) -> (s? t:f=w532:string)
    n298 = call <vilib>:"Delimited String to 1D String Array.vi"("delimiter"=",", "delimited string"=w532) -> ("string array"=w603:string[])  [unwired: 9 in]
    n299 = call "체크섬 문자열 생성기_진최종(SubVI).vi"("raw data 입력"=w543, "GPS ID 입력"="GNGGA," ("GPS ID"), "입력 문자열 입력"=w543, "시프트레지스터(이전값) 입력 입력"=w509) -> ("숫자"=w519:u8, "checksum 확인용 문자열 2"=w542:string, "시프트레지스터용 출력 문자열"=w508:string, "클러스터 분배용 문자열 2"=w515:string, "클러스터 분배용 시프트레지스터"=w505:string)  [unwired: 3 in]
    n300 = call "체크섬 확인(쉼표 포함Ver.).vi"("입력 문자열"=w542) -> ("Checksum 비교값"=w541:u8)  [unwired: 10 in]
    n301 = Equal?(x=w519, y=w541) -> (x = y?=w540:bool)
    n302 = Array To Cluster(array=w603) -> (cluster=w589:T10)
    n303 = Match Pattern(string=w509, regular expression=w508) -> ()  [unwired: 1 in, 4 out]
    n304 = Unbundle(w589) -> ("string array[0]"=w595:string, "string array[1]"=w596:string, "string array[2]"=w597:string, "string array[3]"=w598:string, "string array[4]"=w599:string, "string array[5]"=w600:string, "string array[6]"=w601:string, "string array[7]"=w518:string, "string array[8]"=w517:string)
    n305 = Select(t=w515, s=w540, f=w505) -> (s? t:f=w533:string)
    n306 = call <vilib>:"Delimited String to 1D String Array.vi"("delimiter"=",", "delimited string"=w533) -> ("string array"=w639:string[])  [unwired: 9 in]
    n307 = Array To Cluster(array=w639) -> (cluster=w620:T9)
    n308 = Fract/Exp String To Number(string=w595) -> (number=w565:dbl)  [unwired: 3 in, 1 out]
    n309 = Fract/Exp String To Number(string=w597) -> (number=w592:dbl)  [unwired: 3 in, 1 out]
    n310 = Fract/Exp String To Number(string=w599) -> (number=w593:dbl)  [unwired: 3 in, 1 out]
    n311 = Fract/Exp String To Number(string=w601) -> (number=w594:dbl)  [unwired: 3 in, 1 out]
    n312 = Unbundle(w620) -> ("string array[0]"=w625:string, "string array[1]"=w626:string, "string array[2]"=w627:string, "string array[3]"=w636:string, "string array[4]"=w637:string, "string array[5]"=w628:string, "string array[6]"=w629:string, "string array[7]"=w630:string, "string array[8]"=w631:string, "string array[9]"=w632:string, "string array[10]"=w633:string, "string array[11]"=w634:string, "string array[12]"=w635:string)
    n313 = Fract/Exp String To Number(string=w625) -> (number=w578:dbl)  [unwired: 3 in, 1 out]
    n314 = Fract/Exp String To Number(string=w626) -> (number=w577:dbl)  [unwired: 3 in, 1 out]
    n315 = Fract/Exp String To Number(string=w636) -> (number=w624:dbl)  [unwired: 3 in, 1 out]
    n316 = Fract/Exp String To Number(string=w628) -> (number=w571:dbl)  [unwired: 3 in, 1 out]
    n317 = Fract/Exp String To Number(string=w629) -> (number=w576:dbl)  [unwired: 3 in, 1 out]
    n318 = Fract/Exp String To Number(string=w630) -> (number=w622:dbl)  [unwired: 3 in, 1 out]
    n319 = Fract/Exp String To Number(string=w631) -> (number=w623:dbl)  [unwired: 3 in, 1 out]
    n320 = Bundle(cluster=T4 {"Course"=0.0, "Reference"="", "Course in degrees"=0.0, "Reference"="", "Speed"=0.0, "Unit"="", "Speed"=0.0, "K"="", "A"="", "Checksum"=0}, "Course"=w565, "Reference"=w596, "Course in degrees"=w592, "Reference"=w598, "Speed"=w593, "Unit"=w600, "Speed"=w594, "K"=w518, "A"=w517, "Checksum"=w516) -> (→"VTG":T4)
    n321 = Bundle(cluster=T3 {"UTC time"=0.0, "Latitude"=0.0, "N/S Indicator"="", "Longitude"=0.0, "E/W Indicator"="", "Position FIx"=0, "Satelites Used"=0, "HDOP"=0.0, "Altitude"=0.0, "Altitude Units"="", "empty"="", "empty"="", "empty"="", "Checksum"=0}, "UTC time"=w578, "Latitude"=w577, "N/S Indicator"=w627, "Longitude"=w624, "E/W Indicator"=w637, "Position FIx"=w571, "Satelites Used"=w576, "HDOP"=w622, "Altitude"=w623, "Altitude Units"=w632, "empty"=w633, "empty"=w634, "empty"=w635, "Checksum"=w519) -> (w588:T3)
    "GGA" <- w588
    n322 = Unbundle By Name(w588) -> ("Latitude"=w548:dbl, "Longitude"=w556:dbl, "UTC time"=w557:dbl)
    n323 = To Unsigned Byte Integer(number=w576) -> (unsigned 8bit integer=w575:u8)
    n324 = To Unsigned Byte Integer(number=w571) -> (unsigned 8bit integer=w573:u8)
    n325 = Insert Into Array(array=w584, new element=w556) -> (w587:dbl[])  [unwired: 1 in]
    n326 = Insert Into Array(array=w585, new element=w548) -> (w586:dbl[])  [unwired: 1 in]
    n327 = Format Into String(format string="%d\\t%f\\t%f\\t%f\\t%f\\t\\t%d\\t\\t%f\\t\\t%d\\n" ("포맷 문자열"), initial string=w580, w502, w557, w548, w556, w555, w575, w565, w573) -> (resulting string=w572:refnum<file>)  [unwired: 1 in, 1 out]
    n328 = call "도분초 (SubVI).vi"("구좌표값"=w548) -> ("숫자형"=w547:dbl, "도(*string)"=→"도(Lat)":string, "도분초(string)"=→"도분초(Lat)":string)  [unwired: 8 in]
    n329 = call "도분초 (SubVI).vi"("구좌표값"=w556) -> ("숫자형"=w558:dbl, "도(*string)"=→"도(Long)":string, "도분초(string)"=→"도분초(Long)":string)  [unwired: 8 in]
    n330 = Bundle("배열"=w586, "배열"=w587) -> (→"구좌표플롯":cluster{"배열":dbl[], "배열":dbl[]})  [unwired: 1 in]
    n331 = call "tm_trans.vi"("Long"=w558, "Lat"=w547) -> ("Numeric"=w499:dbl, "out_pt"=w500:dbl)  [unwired: 8 in]
    "Y(E)" <- w500
    "X(N)" <- w499
    n332 = Format Into String(format string="%d\\t%f\\t%f\\n" ("포맷 문자열"), w502, w500, w499) -> ()  [unwired: 2 in, 2 out]
    n333 = Insert Into Array(array=w530, new element=w500) -> (w528:dbl[])  [unwired: 1 in]
    n334 = Insert Into Array(array=w529, new element=w499) -> (w527:dbl[])  [unwired: 1 in]
    n335 = Bundle(w528, w527) -> (→"평면좌표플롯":cluster{dbl[], dbl[]})  [unwired: 1 in]
  }
  n336 = disable-structure shown="비활성화" {
    frame Disabled {
      # "lvcomm.chm::/String_To_IP.html"
      n337 = call "pure pursuit (SubVI).vi"("GPS 헤딩값"="GPS 헤딩값", "축거(m)"="축거(m)", "GPS Y값"="GPS Y값", "Ld"="Ld", "다음wp Y값"="다음wp Y값", "GPS X값"="GPS X값", "다음wp X값"="다음wp X값") -> ("결과 조향값"=→"결과 조향값":dbl)  [unwired: 4 in]
    }
    frame Enabled {
    }
  }
  n338 = Close File(refnum=w21) -> ()  [unwired: 1 in, 2 out]
  n339 = VISA Flush I/O Buffer(VISA resource name=w14, error in (no error)=w13) -> (VISA resource name out=w15:refnum<visa-resource-name>, error out=w16:errorcluster)  [unwired: 1 in]
  n340 = VISA Close(VISA resource name=w15, error in (no error)=w16) -> (error out=→"에러 출력":errorcluster)
  n341 = UDP Close(connection ID=w30) -> ()  [unwired: 1 in, 2 out]
  n342 = disable-structure shown="비활성화" {
    frame Disabled {
      n343 = call "ERP-42 시리얼 통신 (SubVI).vi"("시리얼 루프 정지"="시리얼 루프 정지", "baud rate"="baud rate", "E-Stop"="E-Stop", "timeout (100)"="timeout (100)", "컨트롤러 입력"="transmit Data", "VISA 참조 번호 입력"="시리얼 포트 설정") -> ("Receive Data"=→"Receive Data":T5)  [unwired: 5 in]
    }
    frame Enabled {
    }
  }
